vi "Full front panel (SubVI).vi"(0 "Signal in":dbl[](array[numeric]), 1 "Time in":dbl[](array[numeric]), 2 "Integrate Array":dbl[](array[numeric]), 3 "Path 1":path, 4 "XYGraph Refnum":refnum<vi>, 6 "Boolean":bool[](array[boolean]), 7 "Add element 1":string, 10 "String":refnum<vi>, 11 "Sample list":i32(listbox)=-1, 12 "Sample list 2":refnum<vi>, 13 "mean In":dbl, 16 "Elapsed Time (s)":dbl) -> (5 "Concentrations":dbl[](array[numeric]), 8 "?":cluster{"all rows":dbl[], "all rows":dbl[]}(graph), 9 "Mean":dbl, 14 "Signal out":dbl[](array[numeric]), 15 "Time out":dbl[](array[numeric]), 17 "Plot":cluster{dbl[], dbl[]}(graph), 18 "Current Element":string, 19 "All samples":i32)   [LabVIEW 2014]
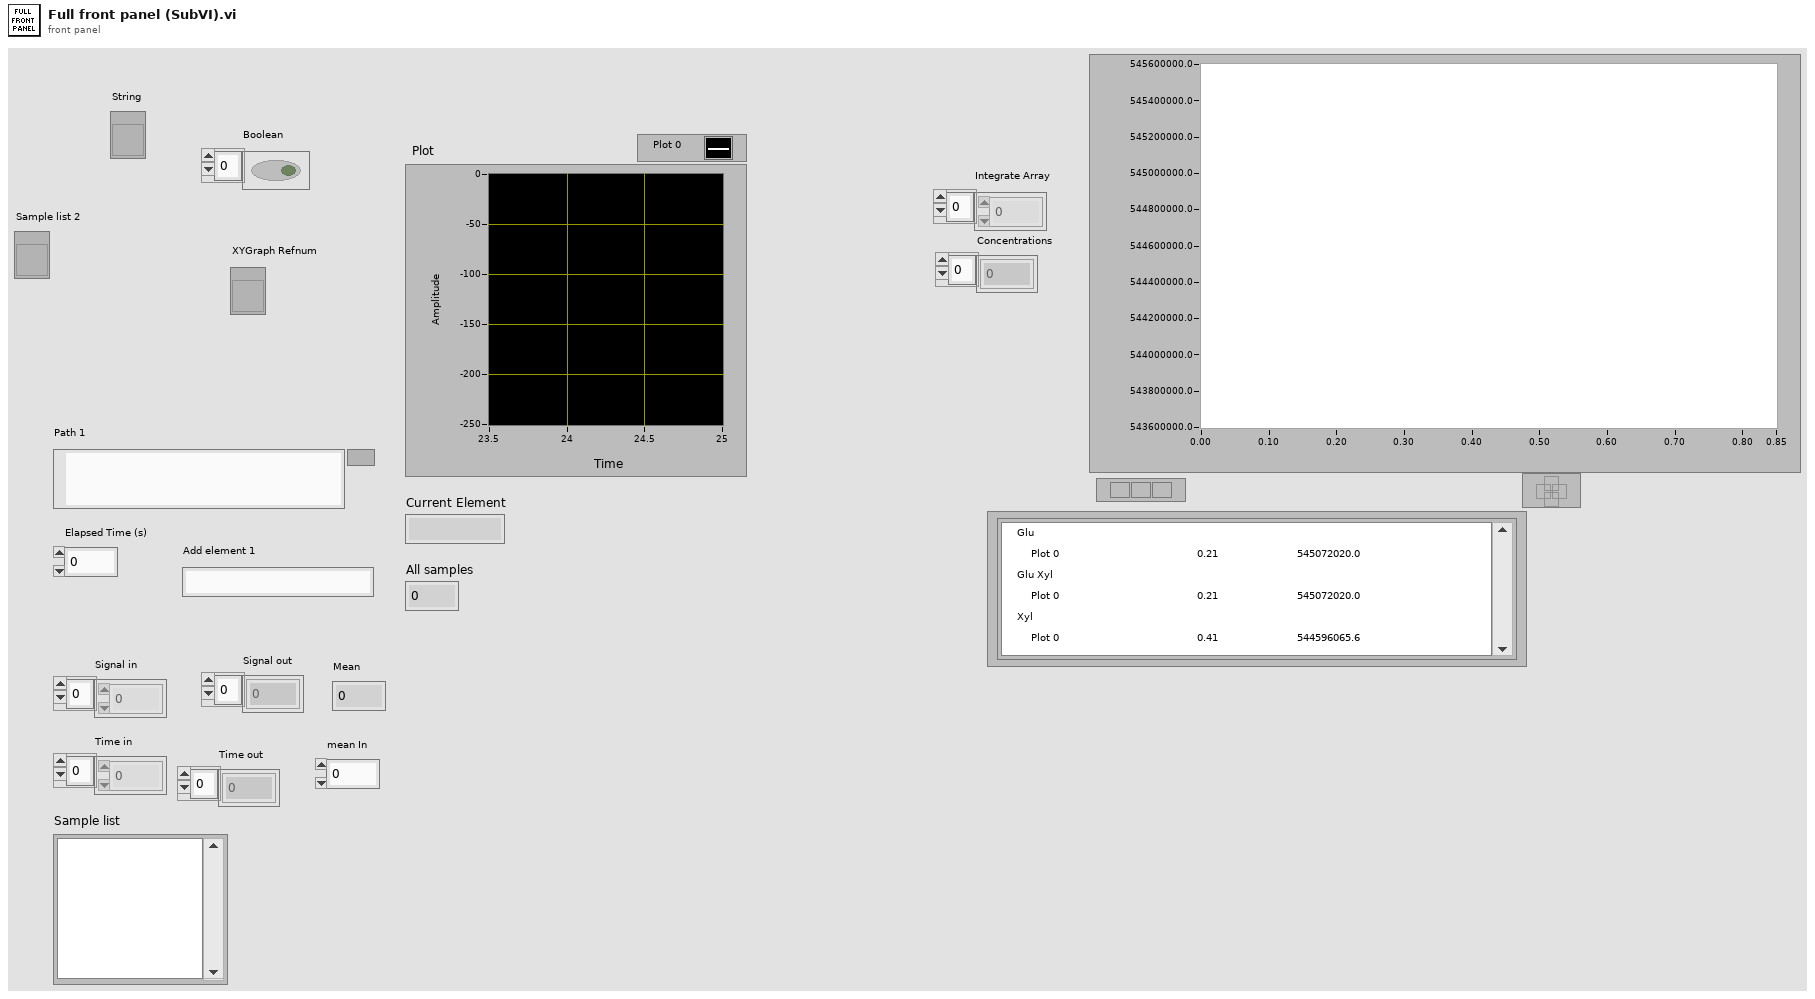
[diagram p1: front panel]
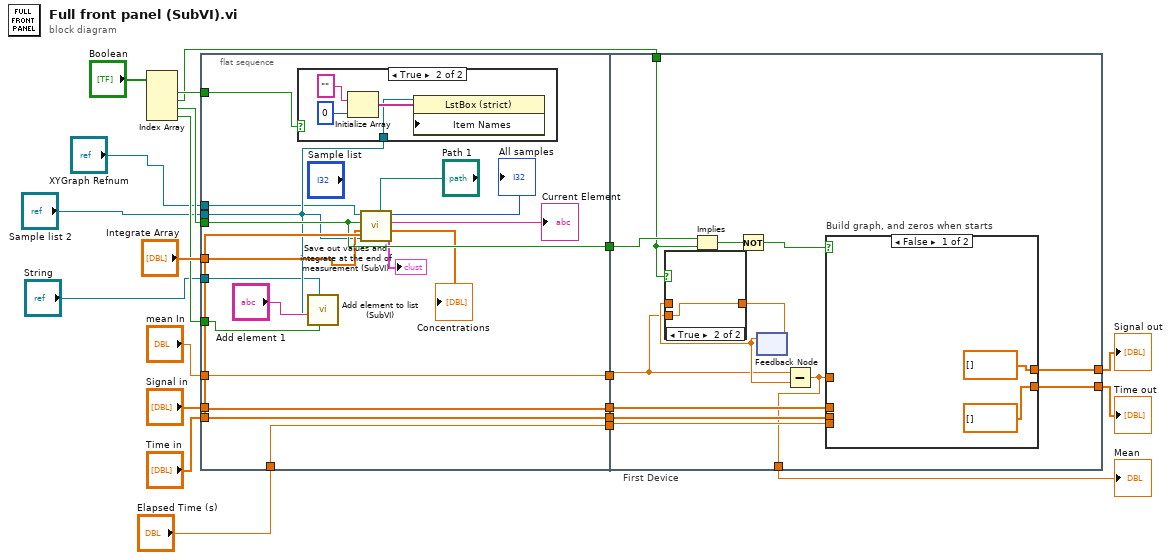
[diagram p0: block diagram]
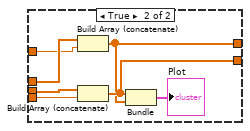
[diagram p4: hidden frame]
diagram:
  n1 = Index Array(array="Boolean") -> (element #1=w7:bool, element #2=w6:bool, element #3=w5:bool, element #4=w4:bool)  [unwired: 4 in]
  n2 = flat-sequence "First Device" {
    tunnel: w5 -> [w31]
    tunnel: "Signal in" -> [w32]
    tunnel: "Time in" -> [w36]
    tunnel: [w32] -> w21
    tunnel: [w36] -> w20
    tunnel: [w30] -> w19
    tunnel: "mean In" -> [w35]
    tunnel: [w35] -> w18
    tunnel: [w31] -> w12
    tunnel: "Elapsed Time (s)" -> [w30]
    tunnel: "Integrate Array" -> [w27]
    tunnel: w7 -> [w26]
    tunnel: w4 -> [w25]
    tunnel: "Sample list 2" -> [w24]
    tunnel: "String" -> [w23]
    tunnel: "XYGraph Refnum" -> [w22]
    tunnel: [w55] -> w16
    tunnel: [w54] -> w17
    tunnel: w21 -> [w53]
    tunnel: w20 -> [w52]
    tunnel: w19 -> [w51]
    tunnel: w18 -> [w48]
    tunnel: w12 -> [w46]
    tunnel: [w47] -> w10
    tunnel: w6 -> [w45]
    frame #0 {
      n3 = case shown="True" w26 {
        tunnel: w24 -> [_ w39]
        frame False {
        }
        frame True {
          n4 = Initialize Array("", 0 ("dimension size")) -> (w42:string[])
          n5 = property on="Property Node" class="LstBox (strict)"(reference=w39, "Item Names"=w42) -> ()  [unwired: 1 in, 2 out]
        }
      }
      n6 = call "Add element to list (SubVI).vi"("Boolean"=w25, "String"=w23, "Add string"="Add element 1", "ListBox in"=w24) -> ()  [unwired: 8 in]
      n7 = call "Save out values and integrate at the end of measurement (SubVI).vi"("Measurement Array"=w32, "Path"="Path 1", "Time Array"=w36, "ListBox in 2"=w24, "Integrate Array"=w27, "Measurement running?"=w31, "XYGraph Refnum"=w22) -> (0:→"?":cluster{"all rows":dbl[], "all rows":dbl[]}, "Concentrations"=→"Concentrations":dbl[], "element"=→"Current Element":string, "size(s)"=→"All samples":i32)  [unwired: 1 in]
    }
    frame #1 {
      n8 = Implies(1:w45, 2:w46) -> (0:w44:bool)
      n9 = Not(x=w44) -> (.not. x?=w43:bool)
      n10 = feedback #1() -> (w49:dbl)  [unwired: 1 in]
      n11 = case shown="True" w45 {
        tunnel: w48 -> [_ w57]
        tunnel: [w56 w57] -> w50
        tunnel: w49 -> [w56 _]
        frame False {
        }
        frame True {
        }
      }
      n12 = feedback-in #1(w50) -> ()
      n13 = Subtract(x=w48, y=w49) -> (x-y=w47:dbl)
      n14 = case "Build graph, and zeros when starts" shown="False" w43 {
        tunnel: [dbl[] [] w64] -> w54
        tunnel: w53 -> [_ w62]
        tunnel: w52 -> [_ w66]
        tunnel: [dbl[] [] w65] -> w55
        tunnel: w51 -> [_ w63]
        tunnel: w47 -> [_ w61]
        frame False {
        }
        frame True {
          n15 = Build Array (concatenate)(w62, w61) -> (w64:dbl[])
          n16 = Build Array (concatenate)(w66, w63) -> (w65:dbl[])
          n17 = Bundle(w65, w64) -> (→"Plot":cluster{dbl[], dbl[]})  [unwired: 1 in]
        }
      }
    }
  }
  "Signal out" <- w17
  "Time out" <- w16
  "Mean" <- w10
